vi "GetTargetPoint.vi"(8 "Pose":T1, 10 "Waypoint Index":dbl, 11 "Waypoints":cluster{"Longitude":dbl, "Latitude":dbl}[](array[cluster])) -> (0 "Close to Waypoint?":bool, 2 "Waypoint Index Out":dbl, 3 "Target Point":cluster{"Target X":dbl, "Target  Y":dbl})   [LabVIEW 2011]
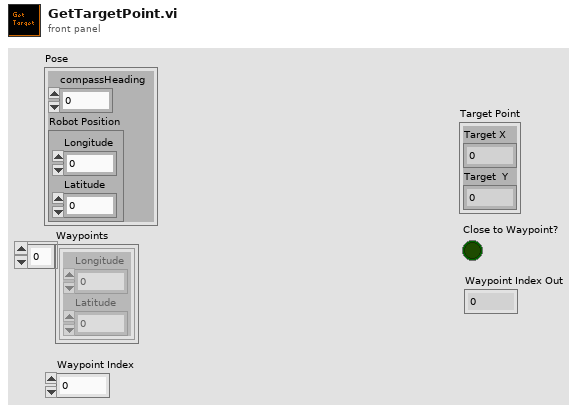
[diagram p1: front panel]
types:
  T1 = cluster{"compassHeading":dbl, "Robot Position":cluster{"Longitude":dbl, "Latitude":dbl}}
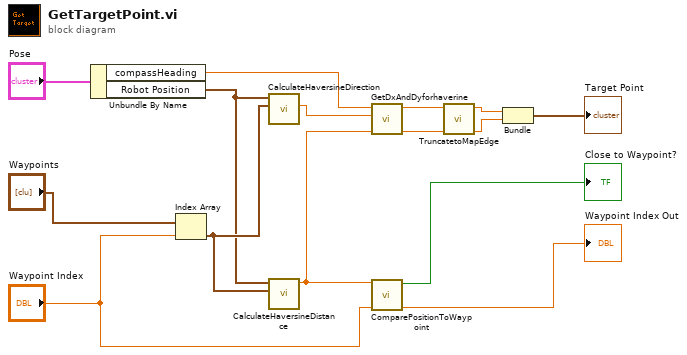
[diagram p0: block diagram]
diagram:
  n1 = Unbundle By Name("Pose") -> ("compassHeading"=w10:dbl, "Robot Position"=w12:cluster{"Longitude":dbl, "Latitude":dbl})
  n2 = Index Array(array="Waypoints", index="Waypoint Index") -> (element=w13:cluster{"Longitude":dbl, "Latitude":dbl})
  n3 = call "CalculateHaversineDirection.vi"("Target Waypoint"=w13, "Robot Position"=w12) -> ("polar angle"=w11:dbl)  [unwired: 9 in]
  n4 = call "CalculateHaversineDistance.vi"("Target Waypoint"=w13, "Robot Position"=w12) -> ("distance (dm)"=w4:dbl)  [unwired: 9 in]
  n5 = call "GetDxAndDyforhaverine.vi"("distance (dm)"=w4, "polar angle"=w11, "compassHeading"=w10) -> ("dx"=w8:dbl, "dy"=w9:dbl)  [unwired: 7 in]
  n6 = call "ComparePositionToWaypoint.vi"("Waypoint Index"="Waypoint Index", "distance (dm)"=w4) -> ("Next Waypoint Index"=→"Waypoint Index Out":dbl, "Close to Waypoint"=→"Close to Waypoint?":bool)  [unwired: 8 in]
  n7 = call "TruncatetoMapEdge.vi"("dx"=w8, "dy"=w9) -> ("Target X"=w6:dbl, "Target Y"=w7:dbl)  [unwired: 8 in]
  n8 = Bundle("Target Y"=w7, "Target X"=w6) -> (→"Target Point":cluster{"Target Y":dbl, "Target X":dbl})  [unwired: 1 in]
